vi "Configure Averaging.vi"(8 "error in (no error)":errorcluster, 9 "Number of Samples (100)":i32=100, 10 "Average State (T: On)":bool=TRUE, 11 "VISA resource name":refnum<visa-resource-name>) -> (0 "error out":errorcluster, 3 "VISA resource name out":refnum<visa-resource-name>)   [LabVIEW 2019, in "Pendulum CNT90.lvlib"]
doc: "Switch on/off the average function and sets the number of samples to use when doing time-interval averaging measurements."
uses:
  Pendulum CNT90.lvlib
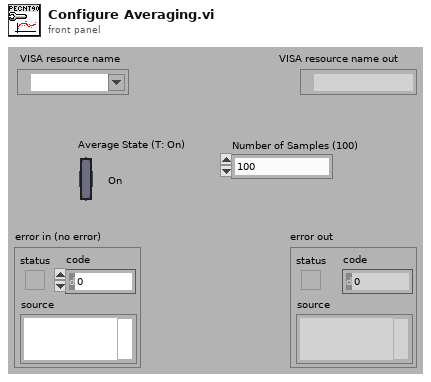
[diagram p1: front panel]
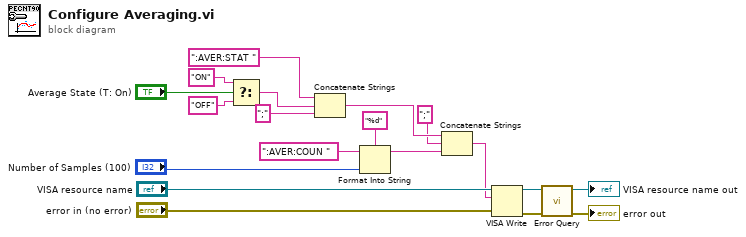
[diagram p0: block diagram]
diagram:
  n1 = Select(t="ON", s="Average State (T: On)", f="OFF") -> (s? t:f=w9:string)
  n2 = Concatenate Strings(":AVER:STAT ", w9, ";" ("string")) -> (w7:string)
  n3 = Format Into String(format string="%d", initial string=":AVER:COUN " ("format string"), "Number of Samples (100)") -> (resulting string=w2:string)  [unwired: 1 in, 1 out]
  n4 = Concatenate Strings(w7, ";" ("string"), w2) -> (w6:string)
  n5 = VISA Write(VISA resource name="VISA resource name", write buffer=w6, error in (no error)="error in (no error)") -> (VISA resource name out=w17:refnum<visa-resource-name>, error out=w14:errorcluster)  [unwired: 1 out]
  n6 = call "Error Query.vi"("error in (no error)"=w14, "VISA resource name"=w17) -> ("error out"=→"error out":errorcluster, "VISA resource name out"=→"VISA resource name out":refnum<visa-resource-name>)  [unwired: 6 in, 2 out]
